vi "Write Limit To Single Line.vi"(8 "error in (no error)":errorcluster, 10 "LimitSglLine":bool, 11 "String.lvclass in":refnum<class "String.lvclass">) -> (0 "error out":errorcluster, 3 "String.lvclass out":refnum<class "String.lvclass">)   [LabVIEW 2015, in "String.lvclass"]
uses:
  String.lvclass
  String.lvclass/String.ctl
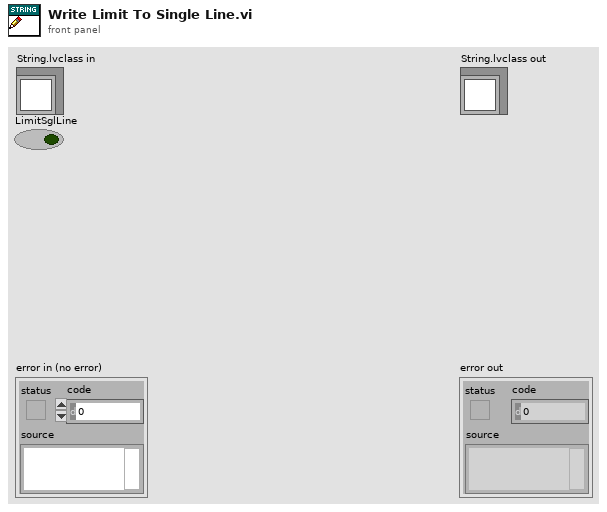
[diagram p1: front panel]
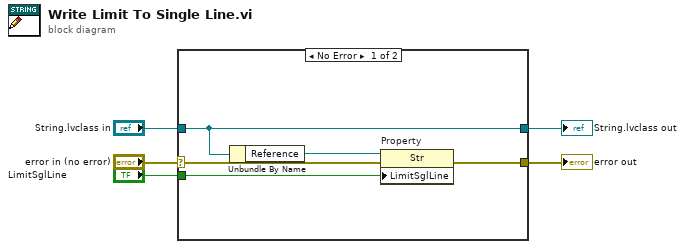
[diagram p0: block diagram]
diagram:
  n1 = case shown="No Error" "error in (no error)" {
    selector: "error in (no error)" -> [w6 w12]
    tunnel: [w10 w12] -> w4
    tunnel: [w8 w11] -> w2
    tunnel: "String.lvclass in" -> [w8 w11]
    tunnel: "LimitSglLine" -> [w9 _]
    frame No Error {
      n2 = Unbundle By Name(w8) -> ("Reference"=w7:refnum<vi>)
      n3 = property on="Property" class="Str"(reference=w7, error in=w6, "LimitSglLine"=w9) -> (error out=w10:errorcluster)  [unwired: 1 out]
    }
    frame Error {
    }
  }
  "error out" <- w4
  "String.lvclass out" <- w2
